vi "Update Energized.vi"(6 "Time":dbl, 8 "error in (no error)":errorcluster, 11 "2WayValve in":refnum<class "2WayValve.lvclass">) -> (0 "error out":errorcluster, 3 "2WayValve out":refnum<class "2WayValve.lvclass">)   [LabVIEW 2020, in "VolatusGUI.lvlib" / "2WayValve.lvclass"]
uses:
  2WayValve.lvclass
  2WayValve.lvclass/2WayValve.ctl
  lv-vecto/Vecto/Channel/Channel.lvclass
  lv-vecto/Vecto/Vecto.lvlib
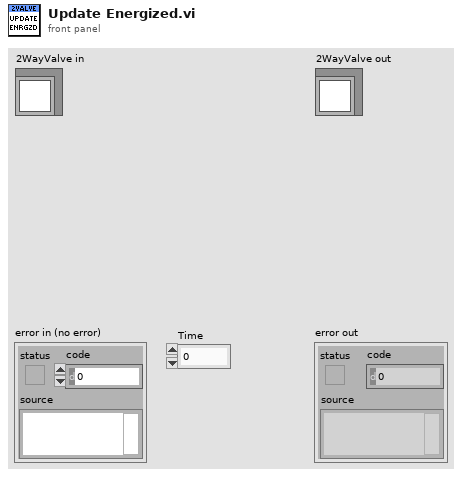
[diagram p1: front panel]
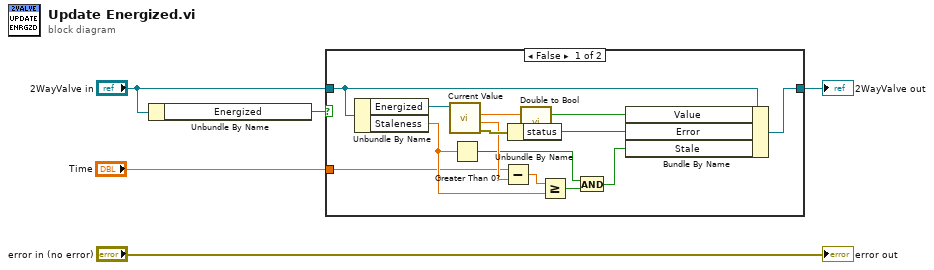
[diagram p0: block diagram]
diagram:
  n1 = Unbundle By Name("2WayValve in") -> ("Energized"=w2:bool)
  n2 = case shown="False" w2 {
    tunnel: [w6 w20] -> w4
    tunnel: "2WayValve in" -> [w7 w20]
    tunnel: "Time" -> [w8 _]
    frame False {
      n3 = Unbundle By Name(w7) -> ("Energized"=w18:refnum<class "Channel.lvclass">, "Staleness"=w12:dbl)
      n4 = call "Current Value.vi"("Channel in"=w18) -> ("error out"=w19:errorcluster, "Timestamp"=w16:dbl, "Scaled"=w17:dbl)  [unwired: 6 in, 2 out]
      n5 = Greater Than 0?(x=w12) -> (x > 0?=w10:bool)
      n6 = Subtract(x=w8, y=w16) -> (x-y=w15:dbl)
      n7 = Unbundle By Name(w19) -> ("status"=w13:bool)
      n8 = call "Double to Bool.vi"("Double"=w17) -> ("Bool"=w14:bool)  [unwired: 2 in]
      n9 = Greater Or Equal?(x=w15, y=w12) -> (x >= y?=w11:bool)
      n10 = And(x=w10, y=w11) -> (x .and. y?=w9:bool)
      n11 = Bundle By Name(cluster=w7, "Value"=w14, "Error"=w13, "Stale"=w9) -> (w6:refnum<class "2WayValve.lvclass">)
    }
    frame True {
      # "Energized Unused"
    }
  }
  "2WayValve out" <- w4
  "error out" <- "error in (no error)"
